vi "conv-V-en-tb.vi"(9 "conf-Aff":T2=[["O"], ["O"], ["O"], ["O"], ["O"], ["O"], ["O"], ["O"], ["O"], ["O"], ["O"], ["O"], ["O"]], 10 "VS":T5, 11 "Etude":T3) -> (0 "do-2D":string[][](array[string]), 1 "ent-2D":T1[][](array[typedef]), 2 "tb in ?":bool[](array[boolean]), 3 "ent tb":T1[](array[typedef]))   [LabVIEW 2010, in "lv_04.lvlib"]
uses:
  lv_04/lv_04.lvlib
  lv_04/commandes/cX.ctl
  lv_04/commandes/cSTA_varid.ctl
  lv_04/commandes/c_TDMS_ch_variable.ctl
  lv_04/commandes/c_TDMS_ch_donnees.ctl
  lv_04/commandes/c0-var-n.ctl
  lv_04/commandes/cSTA_num_do_cr.ctl
  lv_04/commandes/c02-do-num.ctl
  lv_04/commandes/c04-stat-num.ctl
  lv_04/commandes/cSTA_txt_do_cr.ctl
  lv_04/commandes/c02-do-txt.ctl
  lv_04/commandes/c04-stat-txt.ctl
  lv_04/commandes/cSTA_dist.ctl
  lv_04/commandes/c03-dist-S.ctl
  lv_04/commandes/c0-dist-xy.ctl
  lv_04/commandes/c03-dist-T.ctl
  lv_04/commandes/c03-dist-SPC.ctl
  lv_04/commandes/c_etude.ctl
  lv_02/p_5E_ch_loi.ctl
  lv_04/commandes/cSTA-C-config.ctl
  lv_02/lv_02.lvlib
panel:
  out "sous-tableau":string[](array[string])
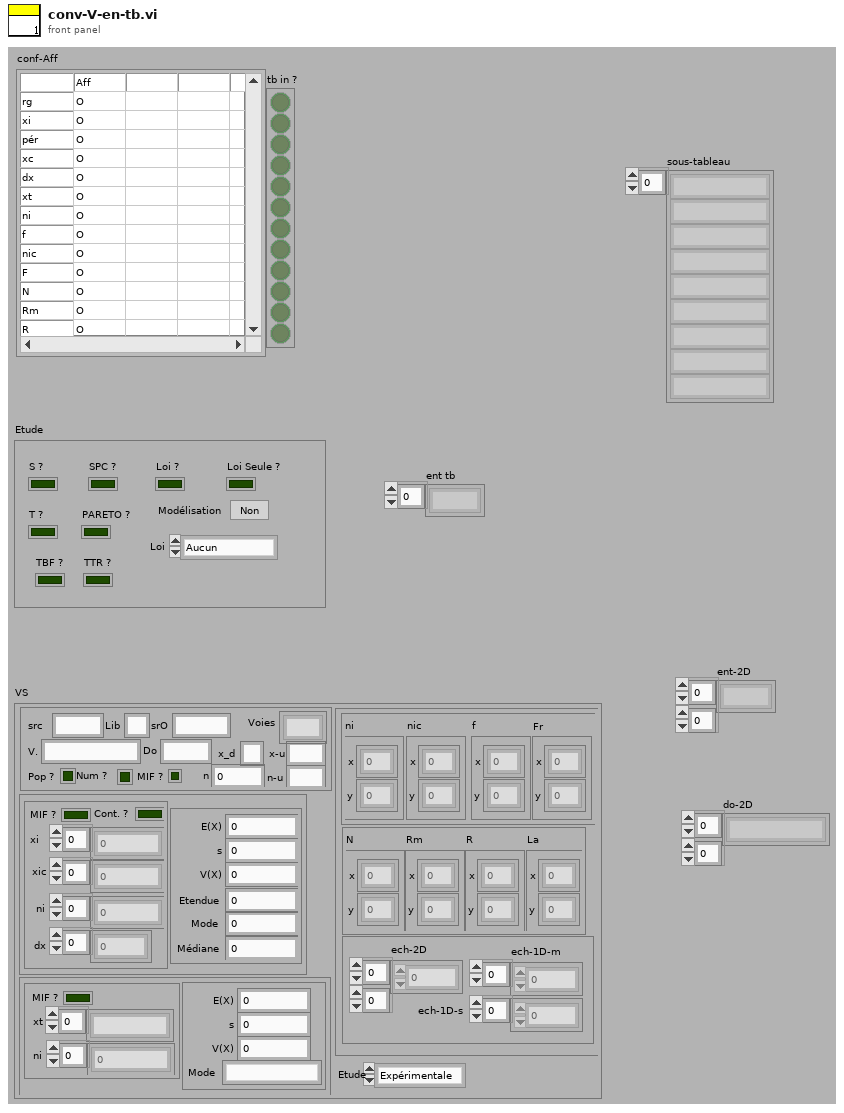
[diagram p1: front panel]
types:
  T1 = typedef "lv_04.lvlib/c_TDMS_ch_donnees.ctl" = string
  T2 = typedef "lv_04.lvlib/cSTA-C-config.ctl" = string[][]
  T3 = typedef "lv_04.lvlib/c_etude.ctl" = cluster{"T ?":bool, "S ?":bool, "SPC ?":bool, "PARETO ?":bool, "TBF ?":bool, "TTR ?":bool, "Loi ?":bool, "Loi Seule ?":bool, "Modélisation":bool, "Loi":T4}
  T4 = typedef "lv_02.lvlib/p_5E_ch_loi.ctl" = enum16{"Aucun", "Normale", "Aucun2", "Aucun3", "Binômial", "Poisson", "Exponentiel", "Weibull", "Rang médian"}
  T5 = typedef "lv_04.lvlib/cX.ctl" = cluster{"src":T6, "num":T9, "txt":T12, "dist":T15, "Etude":enum16{"Expérimentale", "Modèle"}}
  T6 = typedef "lv_04.lvlib/cSTA_varid.ctl" = cluster{"src":string, "Lib":string, "srO":string, "V.":T7, "Voies":string[], "Do":T1, "n":T8, "Num ?":bool, "Pop ?":bool, "x_d":string, "x-u":string, "n-u":string, "MIF ?":bool}
  T7 = typedef "lv_04.lvlib/c_TDMS_ch_variable.ctl" = string
  T8 = typedef "lv_04.lvlib/c0-var-n.ctl" = i32
  T9 = typedef "lv_04.lvlib/cSTA_num_do_cr.ctl" = cluster{"do":T10, "sta":T11}
  T10 = typedef "lv_04.lvlib/c02-do-num.ctl" = cluster{"MIF ?":bool, "Cont. ?":bool, "xi":dbl[], "xic":dbl[], "ni":u32[], "dx":dbl[]}
  T11 = typedef "lv_04.lvlib/c04-stat-num.ctl" = cluster{"E(X)":dbl, "s":dbl, "V(X) ":dbl, "Etendue":dbl, "Mode":dbl, "Médiane":dbl}
  T12 = typedef "lv_04.lvlib/cSTA_txt_do_cr.ctl" = cluster{"do":T13, "sta":T14}
  T13 = typedef "lv_04.lvlib/c02-do-txt.ctl" = cluster{"xt":string[], "ni":dbl[], "MIF ?":bool}
  T14 = typedef "lv_04.lvlib/c04-stat-txt.ctl" = cluster{"E(X)":dbl, "s":dbl, "V(X) ":dbl, "Mode":string}
  T15 = typedef "lv_04.lvlib/cSTA_dist.ctl" = cluster{"S":T16, "T":T18, "spc":T19}
  T16 = typedef "lv_04.lvlib/c03-dist-S.ctl" = cluster{"nic":T17, "f":T17, "Fr":T17, "ni":T17}
  T17 = typedef "lv_04.lvlib/c0-dist-xy.ctl" = cluster{"x":dbl[], "y":dbl[]}
  T18 = typedef "lv_04.lvlib/c03-dist-T.ctl" = cluster{"N":T17, "Rm":T17, "R":T17, "La":T17}
  T19 = typedef "lv_04.lvlib/c03-dist-SPC.ctl" = cluster{"ech-2D":dbl[][], "ech-1D-m":dbl[], "ech-1D-s":dbl[]}
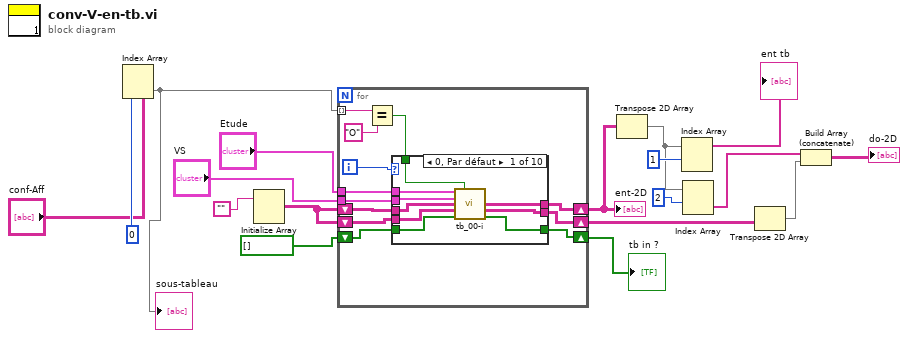
[diagram p0: block diagram]
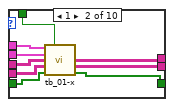
[diagram p2: hidden frame]
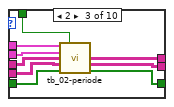
[diagram p3: hidden frame]
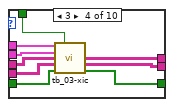
[diagram p4: hidden frame]
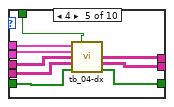
[diagram p5: hidden frame]
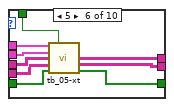
[diagram p6: hidden frame]
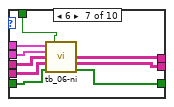
[diagram p7: hidden frame]
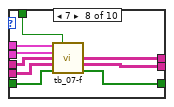
[diagram p8: hidden frame]
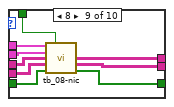
[diagram p9: hidden frame]
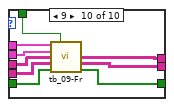
[diagram p10: hidden frame]
diagram:
  n1 = Index Array(array="conf-Aff", index (col)=0 ("indice désactivé (col)")) -> (element=w15:string[])  [unwired: 1 in]
  "sous-tableau" <- w15
  n2 = Initialize Array("") -> (w12:string[][])  [unwired: 2 in]
  n3 = for {
    tunnel: w15 -> [w30] mode=indexing
    tunnel: "VS" -> [w28]
    tunnel: "Etude" -> [w27]
    shift-right: [w22] -> w2
    shift-left: w12 -> [w26]
    shift-right: [w23] -> w5
    shift-left: w12 -> [w25]
    shift-right: [w21] -> w11
    shift-left: bool[] [] ("tb in ? 2") -> [w20]
    i -> [w19]
    n4 = Equal?(x=w30, y="O") -> (x = y?=w24:bool)
    n5 = case shown="0, Par défaut" w19 {
      tunnel: w28 -> [w38 w48 w56 w65 w74 w83 w92 w101 w110 w119]
      tunnel: w27 -> [w39 w47 w57 w66 w75 w84 w93 w102 w111 w120]
      tunnel: w26 -> [w37 w46 w55 w64 w73 w82 w91 w100 w109 w118]
      tunnel: w25 -> [w36 w45 w54 w63 w72 w81 w90 w99 w108 w117]
      tunnel: w24 -> [w32 w41 w49 w60 w67 w76 w85 w94 w103 w112]
      tunnel: [w33 w44 w52 w62 w71 w80 w87 w96 w105 w114] -> w23
      tunnel: [w31 w43 w53 w61 w70 w79 w86 w95 w104 w113] -> w22
      tunnel: [w34 w42 w50 w58 w68 w77 w88 w97 w106 w115] -> w21
      tunnel: w20 -> [w35 w40 w51 w59 w69 w78 w89 w98 w107 w116]
      frame 0, Default {
        n6 = call "tb_00-i.vi"("Etude"=w39, "Aff ?"=w32, "VS"=w38, "ent-2D"=w37, "do-2D"=w36, "tb in ?"=w35) -> ("ent-2D 2"=w31:string[][], "do-2D"=w33:string[][], "tb in ?"=w34:bool[])  [unwired: 2 in, 5 out]
      }
      frame 1 {
        n7 = call "tb_01-x.vi"("Etude"=w47, "Aff ?"=w41, "VS"=w48, "ent-2D"=w46, "do-2D"=w45, "tb in ?"=w40) -> ("ent-2D"=w43:T1[][], "do-2D"=w44:string[][], "tb in ?"=w42:bool[])  [unwired: 2 in, 5 out]
      }
      frame 2 {
        n8 = call "tb_02-periode.vi"("Etude"=w57, "Booléen"=w49, "VS"=w56, "ent-2D"=w55, "do-2D"=w54, "tb in ?"=w51) -> ("ent-2D"=w53:T1[][], "do-2D"=w52:string[][], "tb in ?"=w50:bool[])  [unwired: 2 in, 5 out]
      }
      frame 3 {
        n9 = call "tb_03-xic.vi"("Etude"=w66, "Booléen"=w60, "VS"=w65, "ent-2D"=w64, "do-2D"=w63, "tb in ?"=w59) -> ("ent-2D"=w61:T1[][], "do-2D"=w62:string[][], "tb in ?"=w58:bool[])  [unwired: 2 in, 5 out]
      }
      frame 4 {
        n10 = call "tb_04-dx.vi"("Etude"=w75, "Booléen"=w67, "VS"=w74, "ent-2D"=w73, "do-2D"=w72, "tb in ?"=w69) -> ("ent-2D 2"=w70:string[][], "do-2D"=w71:string[][], "tb in ?"=w68:bool[])  [unwired: 3 in, 4 out]
      }
      frame 5 {
        n11 = call "tb_05-xt.vi"("Etude"=w84, "Aff ?"=w76, "VS"=w83, "ent-2D"=w82, "do-2D"=w81, "tb in ?"=w78) -> ("ent-2D"=w79:T1[][], "do-2D"=w80:string[][], "tb in ?"=w77:bool[])  [unwired: 2 in, 5 out]
      }
      frame 6 {
        n12 = call "tb_06-ni.vi"("Etude"=w93, "Aff ?"=w85, "VS"=w92, "ent-2D"=w91, "do-2D"=w90, "tb in ?"=w89) -> ("ent-2D"=w86:T1[][], "do-2D"=w87:string[][], "tb in ?"=w88:bool[])  [unwired: 2 in, 5 out]
      }
      frame 7 {
        n13 = call "tb_07-f.vi"("Etude"=w102, "Aff ?"=w94, "VS"=w101, "ent-2D"=w100, "do-2D"=w99, "tb in ?"=w98) -> ("ent-2D"=w95:T1[][], "do-2D"=w96:string[][], "tb in ?"=w97:bool[])  [unwired: 2 in, 5 out]
      }
      frame 8 {
        n14 = call "tb_08-nic.vi"("Etude"=w111, "Aff ?"=w103, "VS"=w110, "ent-2D"=w109, "do-2D"=w108, "tb in ?"=w107) -> ("ent-2D"=w104:T1[][], "do-2D"=w105:string[][], "tb in ?"=w106:bool[])  [unwired: 2 in, 5 out]
      }
      frame 9 {
        n15 = call "tb_09-Fr.vi"("Etude"=w120, "Aff ?"=w112, "VS"=w119, "ent-2D"=w118, "do-2D"=w117, "tb in ?"=w116) -> ("ent-2D"=w113:T1[][], "do-2D"=w114:string[][], "tb in ?"=w115:bool[])  [unwired: 2 in, 5 out]
      }
    }
  }
  "ent-2D" <- w2
  "tb in ?" <- w11
  n16 = Transpose 2D Array(2D array=w2) -> (transposed array=w1:T1[][])
  n17 = Index Array(array=w1, index (row)=1 ("indice (ligne)")) -> (element=→"ent tb":T1[])  [unwired: 1 in]
  n18 = Index Array(array=w1, index (row)=2 ("indice (ligne)")) -> (element=w7:T1[])  [unwired: 1 in]
  n19 = Transpose 2D Array(2D array=w5) -> (transposed array=w4:string[][])
  n20 = Build Array (concatenate)(w7, w4) -> (→"do-2D":T1[][])
